vi "19-Manhattan Distance.vi"(11 "Scanner Orientations Relative to Scanner 0":T1(array[cluster])=[{{"Name"=" scanner 15 ---", "Sensor"={"Beacons"=[[-747, -486, -412], [-738, -569, -457], [-689, 659, -426], [-629, -538, -431], [-609, 574, -469], [-567, 658, -522], [349, -584, -782], [352, -544, -666], [384, -640, -624], [531, 820, -584], [601, 763, -473], [670, 759, -677]]}}, "x-translation"=34, "y-translation"=39, "z-translation"=1212, "Rotation"=23}, {{"Name"=" scanner 1 ---", "Sensor"={"Beacons"=[[349, -584, -782], [352, -544, -666], [384, -640, -624], [531, 820, -584], [601, 763, -473], [622, -538, -1810], [638, -430, -1787], [670, 759, -677], [696, 843, -1722], [722, -495, -1668], [740, 862, -1927], [747, 824, -1841]]}}, "x-translation"=-1276, "y-translation"=97, "z-translation"=1275, "Rotation"=19}, {{"Name"=" scanner 19 ---", "Sensor"={"Beacons"=[[-816, 800, 310], [-780, 740, 353], [-700, 873, 335], [-387, -903, 381], [-382, -890, 249], [-369, -772, 414], [355, 790, 421], [468, 864, 533], [470, -559, 544], [474, -502, 534], [579, 799, 416], [652, -594, 511]]}}, "x-translation"=23, "y-translation"=18, "z-translation"=-1148, "Rotation"=1}, {{"Name"=" scanner 3 ---", "Sensor"={"Beacons"=[[-491, -632, 1703], [-488, 584, 1879], [-485, -537, 1774], [-484, -581, 1915], [-459, 634, 1840], [-390, 582, 1976], [406, -862, 1644], [478, 602, 1697], [485, -715, 1666], [507, 636, 1841], [510, 625, 1937], [554, -812, 1696]]}}, "x-translation"=16, "y-translation"=-29, "z-translation"=-2262, "Rotation"=2}, {{"Name"=" scanner 23 ---", "Sensor"={"Beacons"=[[-747, -486, -412], [-738, -569, -457], [-736, 344, -1952], [-729, -481, -1900], [-708, -454, -1841], [-689, 659, -426], [-659, 524, -1932], [-642, 349, -1872], [-629, -538, -431], [-609, 574, -469], [-582, -477, -1853], [-567, 658, -522]]}}, "x-translation"=1232, "y-translation"=-18, "z-translation"=1286, "Rotation"=13}, {{"Name"=" scanner 2 ---", "Sensor"={"Beacons"=[[-2012, -382, -2050], [-1975, -571, -1995], [-1947, -494, -2087], [-1874, 495, -2156], [-1870, 507, -1966], [-1863, 549, -547], [-1863, 450, -408], [-1863, 549, -547], [-1863, 450, -408], [-1851, -878, -503], [-1805, 448, -545], [-1764, 557, -2061], [-1753, -745, -565], [-1638, -832, -487]]}}, "x-translation"=2296, "y-translation"=97, "z-translation"=1318, "Rotation"=16}, {{"Name"=" scanner 4 ---", "Sensor"={"Beacons"=[[-1874, 495, -2156], [-1870, 507, -1966], [-1863, 549, -547], [-1863, 450, -408], [-1863, 549, -547], [-1863, 450, -408], [-1805, 448, -545], [-1764, 557, -2061], [-736, 344, -1952], [-689, 659, -426], [-659, 524, -1932], [-642, 349, -1872], [-609, 574, -469], [-567, 658, -522]]}}, "x-translation"=1152, "y-translation"=-1250, "z-translation"=1236, "Rotation"=17}, {{"Name"=" scanner 9 ---", "Sensor"={"Beacons"=[[-3127, 781, -1763], [-3110, -718, -1707], [-3096, 759, -1689], [-3022, -644, -1627], [-3008, 720, -1776], [-3004, -709, -1789], [-2012, -382, -2050], [-1975, -571, -1995], [-1947, -494, -2087], [-1874, 495, -2156], [-1870, 507, -1966], [-1764, 557, -2061]]}}, "x-translation"=2361, "y-translation"=-82, "z-translation"=2400, "Rotation"=10}, {{"Name"=" scanner 5 ---", "Sensor"={"Beacons"=[[-3179, -650, -3200], [-3169, -678, -3158], [-3007, -613, -3219], [-2871, 402, -2828], [-2725, 394, -2943], [-2689, 402, -2937], [-1748, 827, -3269], [-1703, 790, -3298], [-1681, 715, -3317], [-1618, -639, -3197], [-1540, -593, -3245], [-1539, -691, -3153]]}}, "x-translation"=2394, "y-translation"=-32, "z-translation"=3766, "Rotation"=18}, {{"Name"=" scanner 10 ---", "Sensor"={"Beacons"=[[-2012, -382, -2050], [-1975, -571, -1995], [-1947, -494, -2087], [-1874, 495, -2156], [-1870, 507, -1966], [-1764, 557, -2061], [-1748, 827, -3269], [-1703, 790, -3298], [-1681, 715, -3317], [-1618, -639, -3197], [-1540, -593, -3245], [-1539, -691, -3153], [-736, 344, -1952], [-729, -481, -1900], [-708, -454, -1841], [-659, 524, -1932], [-642, 349, -1872], [-582, -477, -1853]]}}, "x-translation"=1185, "y-translation"=91, "z-translation"=2525, "Rotation"=14}, {{"Name"=" scanner 11 ---", "Sensor"={"Beacons"=[[-3197, -808, -4197], [-3121, -723, -4113], [-3012, -775, -4200], [-2790, 685, -4390], [-2760, 694, -4534], [-2716, 580, -4430], [-2049, 869, -4156], [-2026, 854, -4312], [-2004, 869, -4187], [-1675, -662, -4068], [-1537, -716, -4095], [-1479, -711, -4088]]}}, "x-translation"=2457, "y-translation"=48, "z-translation"=4796, "Rotation"=15}, {{"Name"=" scanner 12 ---", "Sensor"={"Beacons"=[[-3197, -808, -4197], [-3179, -650, -3200], [-3169, -678, -3158], [-3121, -723, -4113], [-3012, -775, -4200], [-3007, -613, -3219], [-1675, -662, -4068], [-1618, -639, -3197], [-1540, -593, -3245], [-1539, -691, -3153], [-1537, -716, -4095], [-1479, -711, -4088]]}}, "x-translation"=2413, "y-translation"=1237, "z-translation"=3623, "Rotation"=12}, {{"Name"=" scanner 13 ---", "Sensor"={"Beacons"=[[-2871, 402, -2828], [-2790, 685, -4390], [-2760, 694, -4534], [-2725, 394, -2943], [-2716, 580, -4430], [-2689, 402, -2937], [-2049, 869, -4156], [-2026, 854, -4312], [-2004, 869, -4187], [-1748, 827, -3269], [-1703, 790, -3298], [-1681, 715, -3317]]}}, "x-translation"=2354, "y-translation"=-1125, "z-translation"=3678, "Rotation"=7}, {{"Name"=" scanner 17 ---", "Sensor"={"Beacons"=[[-3110, -718, -1707], [-3022, -644, -1627], [-3004, -709, -1789], [-2978, -694, -633], [-2915, -541, -578], [-2884, -690, -565], [-2012, -382, -2050], [-1975, -571, -1995], [-1947, -494, -2087], [-1851, -878, -503], [-1753, -745, -565], [-1638, -832, -487]]}}, "x-translation"=2424, "y-translation"=1251, "z-translation"=1267, "Rotation"=8}, {{"Name"=" scanner 6 ---", "Sensor"={"Beacons"=[[-1874, -1903, -877], [-1851, -878, -503], [-1826, -1970, -813], [-1765, -1886, -785], [-1753, -745, -565], [-1638, -832, -487], [-747, -486, -412], [-738, -569, -457], [-629, -538, -431], [-387, -903, 381], [-382, -890, 249], [-369, -772, 414]]}}, "x-translation"=1164, "y-translation"=1250, "z-translation"=-15, "Rotation"=11}, {{"Name"=" scanner 7 ---", "Sensor"={"Beacons"=[[-3110, -718, -1707], [-3084, -1727, -542], [-3079, -1731, -587], [-3041, -1576, -568], [-3037, -1713, -1829], [-3022, -644, -1627], [-3004, -709, -1789], [-2978, -694, -633], [-2967, -1623, -1716], [-2963, -1803, -1706], [-2915, -541, -578], [-2884, -690, -565]]}}, "x-translation"=3490, "y-translation"=1240, "z-translation"=1188, "Rotation"=9}, {{"Name"=" scanner 18 ---", "Sensor"={"Beacons"=[[-3127, 781, -1763], [-3096, 759, -1689], [-3008, 720, -1776], [-2943, 1654, -2939], [-2891, 1556, -2845], [-2878, 1592, -2851], [-2871, 402, -2828], [-2725, 394, -2943], [-2689, 402, -2937], [-1990, 1745, -2929], [-1983, 1748, -3022], [-1896, 1593, -2970], [-1874, 495, -2156], [-1870, 507, -1966], [-1768, 1798, -2040], [-1764, 557, -2061], [-1757, 1897, -2087], [-1748, 827, -3269], [-1746, 1988, -2061], [-1703, 790, -3298], [-1681, 715, -3317]]}}, "x-translation"=2426, "y-translation"=-1264, "z-translation"=2514, "Rotation"=21}, {{"Name"=" scanner 20 ---", "Sensor"={"Beacons"=[[-3205, 1890, -1773], [-3162, 1885, -1675], [-3127, 781, -1763], [-3096, 759, -1689], [-3075, 1828, -1709], [-3008, 720, -1776], [-2895, 829, -560], [-2765, 867, -617], [-2732, 776, -615], [-1874, 495, -2156], [-1870, 507, -1966], [-1863, 549, -547], [-1863, 450, -408], [-1863, 549, -547], [-1863, 450, -408], [-1805, 448, -545], [-1768, 1798, -2040], [-1764, 557, -2061], [-1757, 1897, -2087], [-1746, 1988, -2061], [-1581, 1523, -796], [-1512, 1586, -818], [-1507, 1610, -764]]}}, "x-translation"=2341, "y-translation"=-1264, "z-translation"=1211, "Rotation"=3}, {{"Name"=" scanner 21 ---", "Sensor"={"Beacons"=[[-3084, -1727, -542], [-3079, -1731, -587], [-3041, -1576, -568], [-3037, -1713, -1829], [-2967, -1623, -1716], [-2963, -1803, -1706], [-1874, -1903, -877], [-1826, -1970, -813], [-1765, -1886, -785], [-1701, -1766, -1932], [-1671, -1712, -1945], [-1596, -1837, -1945]]}}, "x-translation"=2307, "y-translation"=2338, "z-translation"=1261, "Rotation"=6}, {{"Name"=" scanner 16 ---", "Sensor"={"Beacons"=[[-3084, -1727, -542], [-3079, -1731, -587], [-3046, -2942, -748], [-3041, -1576, -568], [-3003, -2917, -723], [-2990, -2995, -639], [-1954, -1725, 495], [-1947, -1749, 740], [-1945, -1733, 560], [-1874, -1903, -877], [-1826, -1970, -813], [-1765, -1886, -785], [-1734, -3204, -579], [-1679, -3166, -645], [-1592, -3182, -479]]}}, "x-translation"=2316, "y-translation"=2427, "z-translation"=-3, "Rotation"=4}, {{"Name"=" scanner 8 ---", "Sensor"={"Beacons"=[[-4017, -1987, -893], [-3939, -1962, -814], [-3935, -1945, -871], [-3222, -2844, 552], [-3193, -2827, 689], [-3084, -1727, -542], [-3079, -1731, -587], [-3068, -2793, 624], [-3046, -2942, -748], [-3041, -1576, -568], [-3003, -2917, -723], [-2990, -2995, -639], [-2828, -1912, 728], [-2821, -1787, 709], [-2763, -1993, 720]]}}, "x-translation"=3651, "y-translation"=2454, "z-translation"=-15, "Rotation"=20}, {{"Name"=" scanner 14 ---", "Sensor"={"Beacons"=[[-4037, -2963, 322], [-4034, -3187, -584], [-4030, -3286, -692], [-3997, -3085, 447], [-3980, -3100, -635], [-3976, -3075, 292], [-3222, -2844, 552], [-3193, -2827, 689], [-3068, -2793, 624], [-3046, -2942, -748], [-3003, -2917, -723], [-2990, -2995, -639]]}}, "x-translation"=3533, "y-translation"=3667, "z-translation"=159, "Rotation"=5}, {{"Name"=" scanner 22 ---", "Sensor"={"Beacons"=[[-3197, -808, -4197], [-3179, -650, -3200], [-3169, -678, -3158], [-3121, -723, -4113], [-3012, -775, -4200], [-3007, -613, -3219], [-2871, 402, -2828], [-2790, 685, -4390], [-2760, 694, -4534], [-2725, 394, -2943], [-2716, 580, -4430], [-2689, 402, -2937]]}}, "x-translation"=3623, "y-translation"=-9, "z-translation"=3737, "Rotation"=22}, {{"Name"=" scanner 24 ---", "Sensor"={"Beacons"=[[-4158, 724, -2908], [-4121, 785, -2863], [-4096, 758, -2930], [-3205, 1890, -1773], [-3162, 1885, -1675], [-3127, 781, -1763], [-3096, 759, -1689], [-3075, 1828, -1709], [-3008, 720, -1776], [-2943, 1654, -2939], [-2891, 1556, -2845], [-2878, 1592, -2851], [-2871, 402, -2828], [-2725, 394, -2943], [-2689, 402, -2937]]}}, "x-translation"=3477, "y-translation"=-1147, "z-translation"=2567, "Rotation"=13}, {{"Name"=" scanner 25 ---", "Sensor"={"Beacons"=[[-3084, -1727, -542], [-3079, -1731, -587], [-3041, -1576, -568], [-2978, -694, -633], [-2915, -541, -578], [-2884, -690, -565], [-2828, -1912, 728], [-2821, -1787, 709], [-2763, -1993, 720], [-1996, -441, 546], [-1973, -499, 333], [-1954, -1725, 495], [-1947, -1749, 740], [-1945, -1733, 560], [-1913, -396, 424], [-1874, -1903, -877], [-1851, -878, -503], [-1826, -1970, -813], [-1765, -1886, -785], [-1753, -745, -565], [-1638, -832, -487]]}}, "x-translation"=2306, "y-translation"=1164, "z-translation"=-24, "Rotation"=17}, {{"Name"="", "Sensor"={"Beacons"=[]}}, "x-translation"=0, "y-translation"=0, "z-translation"=0, "Rotation"=0}]) -> (3 "max manhattan distancce":i32)   [LabVIEW 2019, in "19.lvlib"]
uses:
  19.lvlib
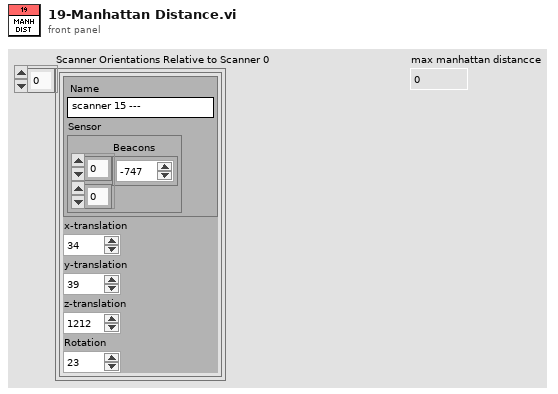
[diagram p1: front panel]
types:
  T1 = cluster{cluster{"Name":string, "Sensor":cluster{"Beacons":i32[][]}}, "x-translation":i32, "y-translation":i32, "z-translation":i32, "Rotation":i32}[]
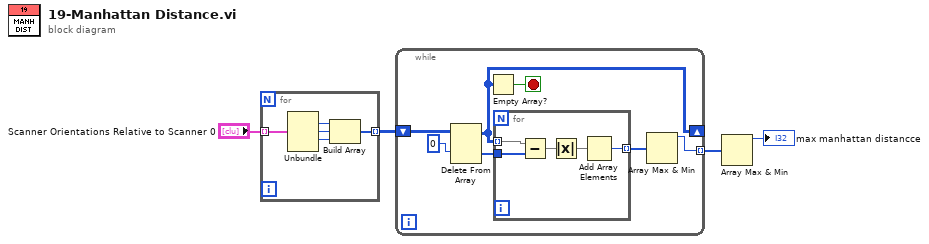
[diagram p0: block diagram]
diagram:
  n1 = for {
    tunnel: "Scanner Orientations Relative to Scanner 0" -> [w9] mode=indexing
    tunnel: [w5] -> w2 mode=indexing
    n2 = Unbundle(w9) -> ("x-translation"=w7:i32, "y-translation"=w6:i32, "z-translation"=w8:i32)  [unwired: 2 out]
    n3 = Build Array(w7, w6, w8) -> (w5:i32[])
  }
  n4 = while {
    shift-right: [w11] -> _
    shift-left: w2 -> [w16]
    tunnel: [w12] -> w4 mode=indexing
    stop <- w10 stop-if-true
    n5 = Delete From Array(array=w16, index (row)=0) -> (deleted portion=w14:i32[], array with subset deleted=w11:i32[][])  [unwired: 2 in]
    n6 = Empty Array?(array=w11) -> (empty?=w10:bool)
    n7 = for {
      tunnel: w11 -> [w20] mode=indexing
      tunnel: w14 -> [w21]
      tunnel: [w17] -> w13 mode=indexing
      n8 = Subtract(x=w20, y=w21) -> (x-y=w19:i32[])
      n9 = Absolute Value(x=w19) -> (abs(x)=w18:i32[])
      n10 = Add Array Elements(numeric array=w18) -> (sum=w17:i32)
    }
    n11 = Array Max & Min(array=w13) -> (max value=w12:i32)  [unwired: 3 out]
  }
  n12 = Array Max & Min(array=w4) -> (max value=→"max manhattan distancce":i32)  [unwired: 3 out]
